vi "KundtsTube.vi"() -> ()   [LabVIEW 2015]
panel:
  in  "Pts":dbl
  in  "Spacing":u16(ring) items=["Linear", "Logorithmic"]
  in  "Max":dbl
  in  "Min":dbl
  out "RMS":dbl
  out "Waveform Graph":dynamicdata(graph)
  in  "# of Samples":dbl
  in  "Sampling Rate":dbl
  in  "Amplitude":dbl
  in  "Frequency":dbl
  in  "Boolean":bool
  in  "Tab Control":enum32{"Sweep ", "Single"}(tab)
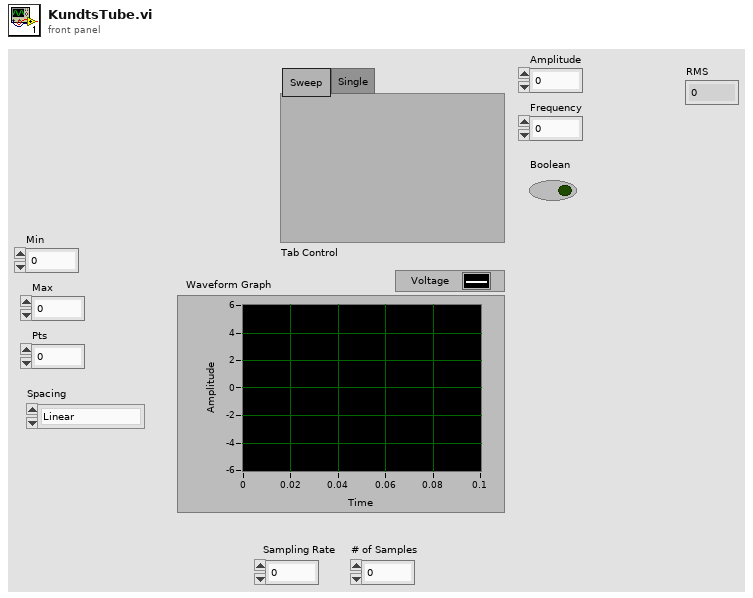
[diagram p1: front panel]
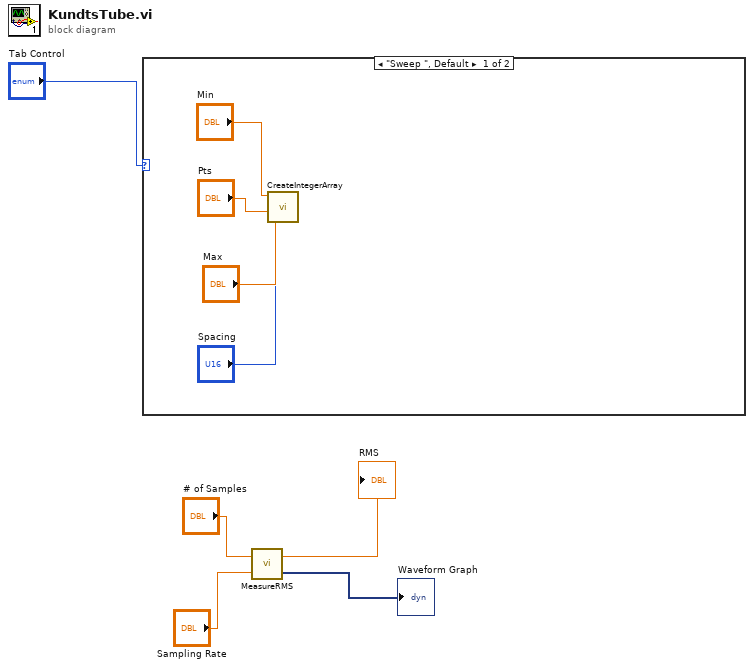
[diagram p0: block diagram]
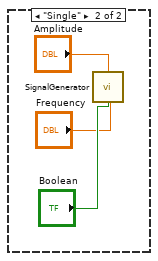
[diagram p2: hidden frame]
diagram:
  n1 = case shown="\"Sweep \", Default" "Tab Control" {
    frame "Sweep ", Default {
      n2 = call "CreateIntegerArray.vi"("Spacing"="Spacing", "Pts"="Pts", "Max"="Max", "Min"="Min") -> ()  [unwired: 1 out]
    }
    frame "Single" {
      n3 = call "SignalGenerator.vi"("Boolean"="Boolean", "Frequency"="Frequency", "Amplitude"="Amplitude") -> ()
    }
  }
  n4 = call "MeasureRMS.vi"("Sampling Rate"="Sampling Rate", "# of Samples"="# of Samples") -> ("Waveform Graph"=→"Waveform Graph":dynamicdata, "RMS"=→"RMS":dbl)
